vi "FTW-CodeGen-SelectMenu5.vi"(0 "State In":T2, 5 "XRef":refnum<vi>, 7 "Tag":string, 9 "Point":cluster{"H":i32, "V":i32}, 11 "Menu Type":T3(ring)) -> (4 "State Out":T2, 6 "Handled?":bool, 8 "Multi Object Popup Options":T1, 10 "Reply":string[](array[string]))   [LabVIEW 2014, in "FTW-Sync-Synchronizer.xnode"]
uses:
  FTW-Sync-Synchronizer.xnode
  FTW-CodeGen-State.ctl
  codegen/FTW-CodeGen-XNodeReplyType.ctl
panel:
  # "Inputs"
  # "Outputs"
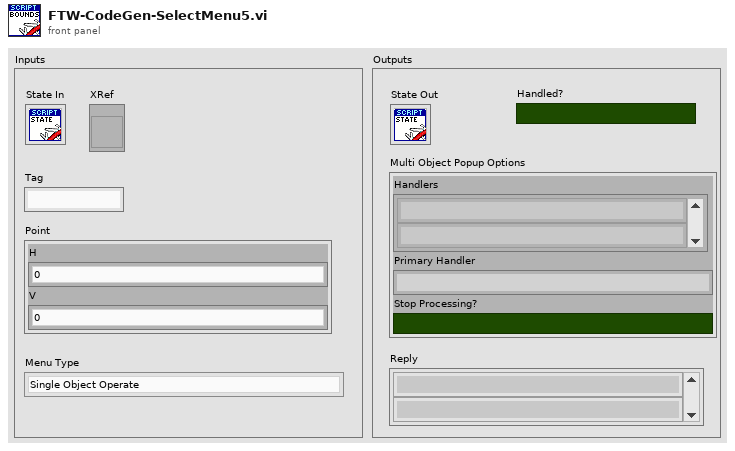
[diagram p1: front panel]
types:
  T1 = cluster{"Handlers":string[], "Primary Handler":string, "Stop Processing?":bool}
  T2 = typedef "FTW-Sync-Synchronizer.xnode/FTW-CodeGen-State.ctl" = cluster{"InputTerminals":cluster{"Wired?":bool, "ID":string, "DataName":string, "DataColor":u32, "Type":variant}[], "EnableTiming?":bool}
  T3 = enum32{"Single Object Operate", "Single Object Popup", "Multi Object Popup Master", "Multi Object Popup Other"}
  T4 = typedef "FTW-CodeGen-XNodeReplyType.ctl" = enum16{"UpdateState", "AdaptToInputs", "AdaptAndAugment", "CosmeticUpdate", "NoReply"}
  T5 = cluster{"Wired?":bool, "ID":string, "DataName":string, "DataColor":u32, "Type":variant}[]
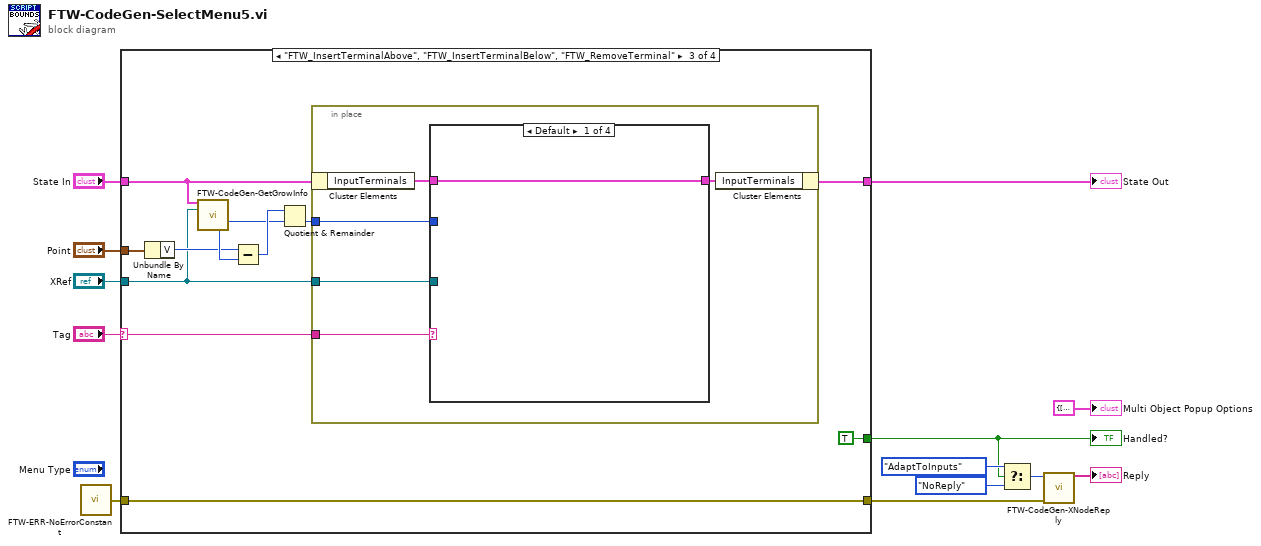
[diagram p0: block diagram]
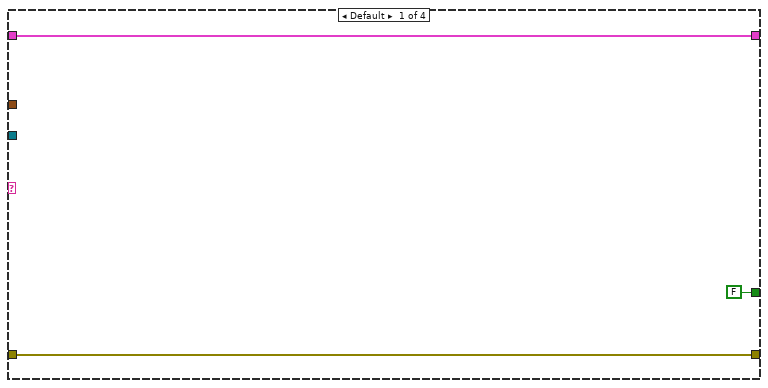
[diagram p2: hidden frame]
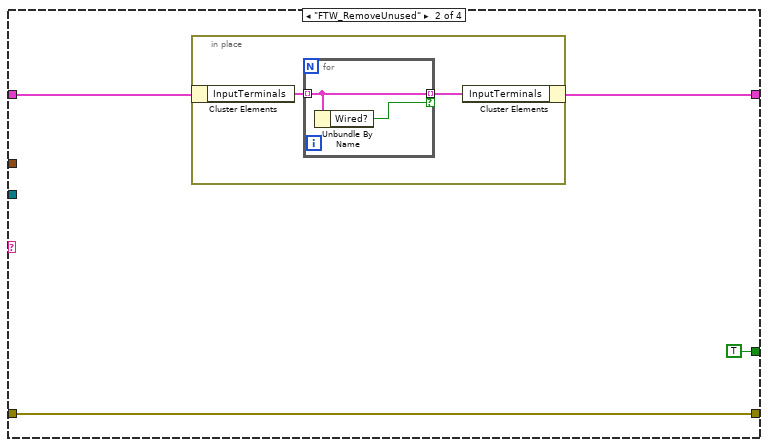
[diagram p3: hidden frame]
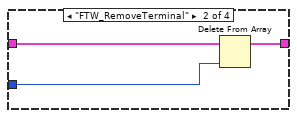
[diagram p4: hidden frame]
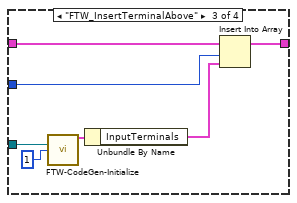
[diagram p5: hidden frame]
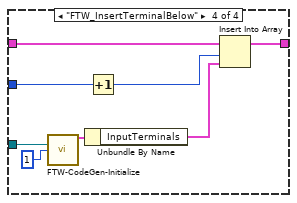
[diagram p6: hidden frame]
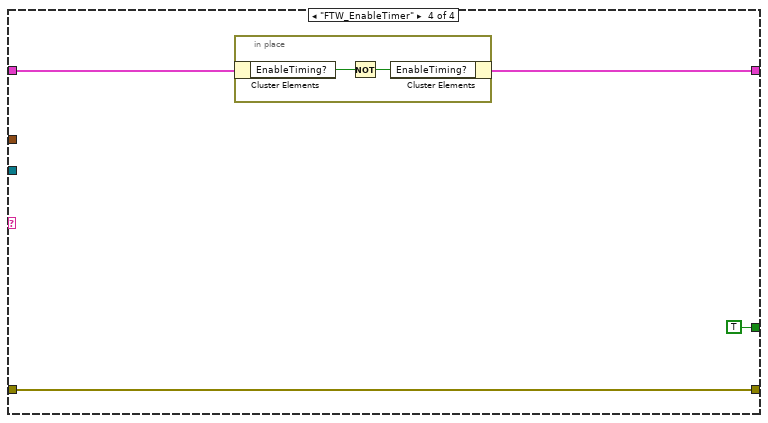
[diagram p7: hidden frame]
diagram:
  n1 = call "FTW-ERR-NoErrorConstant.vi"() -> ("no error"=w6:errorcluster)
  n2 = case shown="\"FTW_InsertTerminalAbove\", \"FTW_InsertTerminalBelow\", \"FTW_RemoveTerminal\"" "Tag" {
    selector: "Tag" -> [_ _ w26 _]
    tunnel: "XRef" -> [_ _ w25 _]
    tunnel: "State In" -> [w16 w20 w29 w63]
    tunnel: "Point" -> [_ _ w33 _]
    tunnel: [w16 w19 w28 w62] -> w8
    tunnel: w6 -> [w15 w17 w31 w61]
    tunnel: [w15 w17 w31 w61] -> w5
    tunnel: [FALSE ("Handled?") TRUE ("Handled?") TRUE ("Handled?") TRUE ("Handled?")] -> w2
    frame Default {
    }
    frame "FTW_RemoveUnused" {
      n3 = in-place {
        n4 = in-place-cluster #1(w20) -> ("InputTerminals"=w22:T5)
        n5 = for {
          tunnel: w22 -> [w24] mode=indexing
          tunnel: [w24] -> w21 mode=indexing if=w23
          n6 = Unbundle By Name(w24) -> ("Wired?"=w23:bool)
        }
        n7 = in-place-cluster #1("InputTerminals"=w21) -> (w19:T2)
      }
    }
    frame "FTW_InsertTerminalAbove", "FTW_InsertTerminalBelow", "FTW_RemoveTerminal" {
      n8 = Unbundle By Name(w33) -> ("V"=w32:i32)
      n9 = call "FTW-CodeGen-GetGrowInfo.vi"("State In"=w29, "XRef"=w25) -> ("Terminal Height"=w34:i32, "Total Top Banner Height"=w36:i32)  [unwired: 5 in, 7 out]
      n10 = Subtract(x=w32, y=w36) -> (x-y=w35:i32)
      n11 = Quotient & Remainder(x=w35, y=w34) -> (floor(x/y)=w27:i32)  [unwired: 1 out]
      n12 = in-place {
        in-place-border: w27 -> [w37]
        in-place-border: w26 -> [w39]
        in-place-border: w25 -> [w38]
        n13 = in-place-cluster #2(w29) -> ("InputTerminals"=w41:T5)
        n14 = case shown="Default" w39 {
          tunnel: w41 -> [w42 w45 w51 w59]
          tunnel: [w42 w44 w50 w58] -> w40
          tunnel: w38 -> [_ _ w49 w57]
          tunnel: w37 -> [_ w43 w47 w55]
          frame Default {
          }
          frame "FTW_RemoveTerminal" {
            n15 = Delete From Array(array=w45, index=w43) -> (array with subset deleted=w44:T5)  [unwired: 1 in, 1 out]
          }
          frame "FTW_InsertTerminalAbove" {
            n16 = call "FTW-CodeGen-Initialize.vi"("XRef"=w49, "Items"=1) -> ("State Out"=w52:T2)  [unwired: 13 in]
            n17 = Unbundle By Name(w52) -> ("InputTerminals"=w46:T5)
            n18 = Insert Into Array(array=w51, index=w47, new element=w46) -> (w50:T5)
          }
          frame "FTW_InsertTerminalBelow" {
            n19 = call "FTW-CodeGen-Initialize.vi"("XRef"=w57, "Items"=1) -> ("State Out"=w60:T2)  [unwired: 13 in]
            n20 = Unbundle By Name(w60) -> ("InputTerminals"=w54:T5)
            n21 = Increment(x=w55) -> (x+1=w53:i32)
            n22 = Insert Into Array(array=w59, index=w53, new element=w54) -> (w58:T5)
          }
        }
        n23 = in-place-cluster #2("InputTerminals"=w40) -> (w28:T2)
      }
    }
    frame "FTW_EnableTimer" {
      n24 = in-place {
        n25 = in-place-cluster #3(w63) -> ("EnableTiming?"=w66:bool)
        n26 = Not(x=w66) -> (.not. x?=w65:bool)
        n27 = in-place-cluster #3("EnableTiming?"=w65) -> (w62:T2)
      }
    }
  }
  "State Out" <- w8
  "Handled?" <- w2
  n28 = Select(t=FTW-CodeGen-XNodeReplyType."AdaptToInputs" ("XNode Reply Type"), s=w2, f=FTW-CodeGen-XNodeReplyType."NoReply" ("XNode Reply Type")) -> (s? t:f=w1:T4)
  n29 = call "FTW-CodeGen-XNodeReply.vi"("XNode Reply Type"=w1, "error in"=w5) -> ("Reply"=→"Reply":string[])  [unwired: 13 in]
  "Multi Object Popup Options" <- T1 {"Handlers"=[], "Primary Handler"="", "Stop Processing?"=FALSE} ("Multi Object Popup Options")
